vi "Get Plugin Paths.vi"(8 "error in":errorcluster, 11 "measurement plugin in":refnum<class "Automotive Ethernet Bus Monitor.lvclass">) -> (0 "error out":errorcluster, 2 "plugin paths":T1, 3 "measurement plugin out":refnum<class "Automotive Ethernet Bus Monitor.lvclass">)   [LabVIEW 2025, in "Automotive Ethernet Bus Monitor.lvclass"]
uses:
  Automotive Ethernet Bus Monitor.lvclass
  <vilib>/Plug-In SDKs/Measurements/Measurement Plugin Service/Plugin Paths.ctl
  Measurement Configuration.ctl
  Measurement Results.ctl
  Measurement Logic.vi
  <vilib>/Plug-In SDKs/Measurements/Measurement Plugin Service/Measurement Plugin Service.lvclass
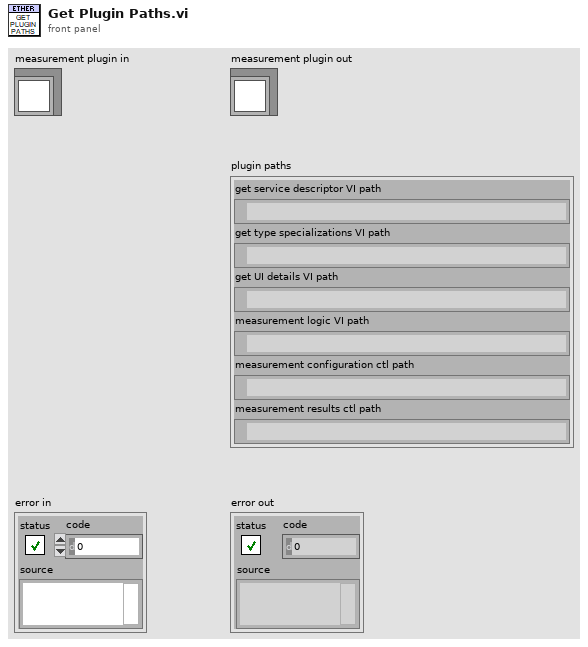
[diagram p1: front panel]
types:
  T1 = typedef "NI Measurement Plug-In SDK.lvlib/Measurement Plugin Service.lvclass/Plugin Paths.ctl" = cluster{"get service descriptor VI path":path, "get type specializations VI path":path, "get UI details VI path":path, "measurement logic VI path":path, "measurement configuration ctl path":path, "measurement results ctl path":path}
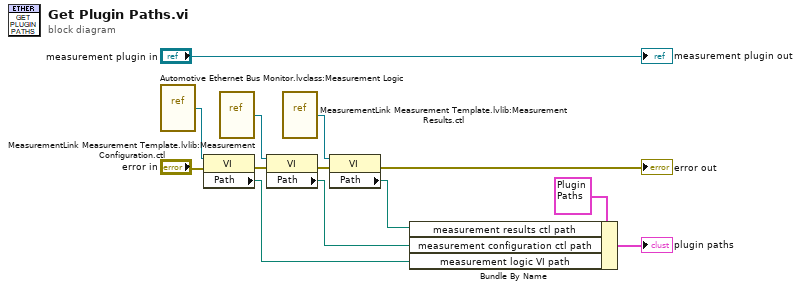
[diagram p0: block diagram]
diagram:
  n1 = vi-ref "Automotive Ethernet Bus Monitor.lvclass:Measurement Logic.vi"() -> (w1:refnum<vi>)
  n2 = property class="VI"(reference=w1, error in="error in") -> (error out=w3:errorcluster, "Path"=w6:path)  [unwired: 1 out]
  n3 = vi-ref "MeasurementLink Measurement Template.lvlib:Measurement Configuration.ctl"() -> (w12:refnum<vi>)
  n4 = property class="VI"(reference=w12, error in=w3) -> (error out=w10:errorcluster, "Path"=w5:path)  [unwired: 1 out]
  n5 = vi-ref "MeasurementLink Measurement Template.lvlib:Measurement Results.ctl"() -> (w11:refnum<vi>)
  n6 = property class="VI"(reference=w11, error in=w10) -> (error out=→"error out":errorcluster, "Path"=w4:path)  [unwired: 1 out]
  n7 = Bundle By Name(cluster=T1 {"get service descriptor VI path"=path "", "get type specializations VI path"=path "", "get UI details VI path"=path "", "measurement logic VI path"=path "", "measurement configuration ctl path"=path "", "measurement results ctl path"=path ""} ("Plugin Paths"), "measurement results ctl path"=w4, "measurement configuration ctl path"=w5, "measurement logic VI path"=w6) -> (→"plugin paths":T1)
  "measurement plugin out" <- "measurement plugin in"
